vi "DUAL GAUGE-TREE.VI"   [LabVIEW 2010, in "Dual Gauge.lvlib"]
uses:
  Dual Gauge.lvlib
panel:
  # "SEE DIAGRAM FOR VI TREE"
  # "Pfeiffer Vacuum GmbH\n Berlinerstrasse 43\n D-35614 Asslar\n\n Telefon +49-6441/802-0\n Telefax +49-6441/802-202\n Internet: http://www.pfeiffer-vacuum.de"
  # "TPG 252\nTPG 261\nTPG 262"
  # "07.01.2001 FPF"
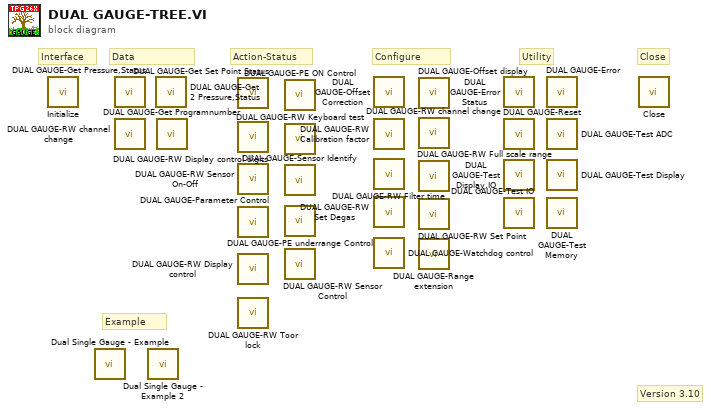
[diagram p0: block diagram]
diagram:
  # "Close"
  # "Example"
  # "Version 3.10"
  # "Utility"
  # "Configure"
  # "Action-Status"
  # "Data"
  # "Interface"
  n1 = call "Initialize.vi"() -> ()  [unwired: 10 in, 2 out]
  n2 = call "Dual Single Gauge - Example.vi"() -> ()  [unwired: 7 in, 5 out]
  n3 = call "DUAL GAUGE-Get Pressure,Status.vi"() -> ()  [unwired: 8 in, 4 out]
  n4 = call "DUAL GAUGE-RW channel change.vi"() -> ()  [unwired: 9 in, 3 out]
  n5 = call "Dual Single Gauge - Example 2.vi"() -> ()  [unwired: 7 in, 5 out]
  n6 = call <instrlib>:"DUAL GAUGE-Get 2 Pressure,Status.vi"() -> ()  [unwired: 6 in, 6 out]
  n7 = call "DUAL GAUGE-Get Programnumber.vi"() -> ()  [unwired: 9 in, 3 out]
  n8 = call "DUAL GAUGE-Get Set Point Status.vi"() -> ()  [unwired: 6 in, 6 out]
  n9 = call "DUAL GAUGE-RW Display control digits.vi"() -> ()  [unwired: 9 in, 3 out]
  n10 = call "DUAL GAUGE-RW Sensor On-Off.vi"() -> ()  [unwired: 12 in, 4 out]
  n11 = call "DUAL GAUGE-Parameter Control.vi"() -> ()  [unwired: 9 in, 3 out]
  n12 = call "DUAL GAUGE-RW Display control.vi"() -> ()  [unwired: 9 in, 3 out]
  n13 = call "DUAL GAUGE-RW Toor lock.vi"() -> ()  [unwired: 9 in, 3 out]
  n14 = call "DUAL GAUGE-PE ON Control.vi"() -> ()  [unwired: 8 in, 4 out]
  n15 = call "DUAL GAUGE-RW Keyboard test.vi"() -> ()  [unwired: 6 in, 6 out]
  n16 = call "DUAL GAUGE-Sensor Identify.vi"() -> ()  [unwired: 8 in, 4 out]
  n17 = call "DUAL GAUGE-PE underrange Control.vi"() -> ()  [unwired: 8 in, 4 out]
  n18 = call "DUAL GAUGE-RW Sensor Control.vi"() -> ()  [unwired: 14 in, 6 out]
  n19 = call "DUAL GAUGE-Offset Correction.vi"() -> ()  [unwired: 8 in, 4 out]
  n20 = call "DUAL GAUGE-RW Calibration factor.vi"() -> ()  [unwired: 8 in, 4 out]
  n21 = call "DUAL GAUGE-RW Filter time.vi"() -> ()  [unwired: 8 in, 4 out]
  n22 = call "DUAL GAUGE-RW Set Degas.vi"() -> ()  [unwired: 8 in, 4 out]
  n23 = call "DUAL GAUGE-Watchdog control.vi"() -> ()  [unwired: 9 in, 3 out]
  n24 = call "DUAL GAUGE-Offset display.vi"() -> ()  [unwired: 8 in, 4 out]
  n25 = call "DUAL GAUGE-RW channel change.vi"() -> ()  [unwired: 9 in, 3 out]
  n26 = call "DUAL GAUGE-RW Full scale range.vi"() -> ()  [unwired: 8 in, 4 out]
  n27 = call "DUAL GAUGE-RW Set Point.vi"() -> ()  [unwired: 15 in, 5 out]
  n28 = call "DUAL GAUGE-Range extension.vi"() -> ()  [unwired: 8 in, 4 out]
  n29 = call "DUAL GAUGE-Error Status.vi"() -> ()  [unwired: 8 in, 4 out]
  n30 = call "DUAL GAUGE-Reset.vi"() -> ()  [unwired: 9 in, 3 out]
  n31 = call "DUAL GAUGE-Test Display,IO.vi"() -> ()  [unwired: 10 in, 2 out]
  n32 = call "DUAL GAUGE-Test IO.vi"() -> ()  [unwired: 8 in, 4 out]
  n33 = call "DUAL GAUGE-Error.vi"() -> ()  [unwired: 9 in, 2 out]
  n34 = call "DUAL GAUGE-Test ADC.vi"() -> ()  [unwired: 6 in, 6 out]
  n35 = call "DUAL GAUGE-Test Display.vi"() -> ()  [unwired: 9 in, 3 out]
  n36 = call "DUAL GAUGE-Test Memory.vi"() -> ()  [unwired: 8 in, 4 out]
  n37 = call "Close.vi"() -> ()  [unwired: 11 in, 1 out]
